vi "Empty Logging Configuration.vi"() -> (0 "Logging Configuration":T1)   [LabVIEW 2021, in "Logging.lvlib"]
doc: "(inline VI) Return an empty Logging Configuration. Use in-place of a block diagram constant.\n\nA cluster representing the settings for the data log file."
uses:
  Logging.lvlib
  Logging Configuration.ctl
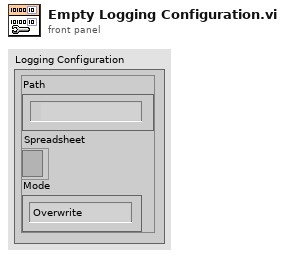
[diagram p1: front panel]
types:
  T1 = typedef "Logging.lvlib/Logging Configuration.ctl" = cluster{"Path":path, "Spreadsheet":refnum<file>, "Mode":enum16{"Overwrite", "Append", "Create New"}}
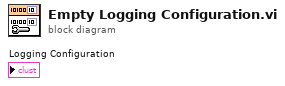
[diagram p0: block diagram]
diagram:
